vi "Constants.vi"   [LabVIEW 2017, in "DSF Core.lvlib"]
uses:
  DSF Core.lvlib
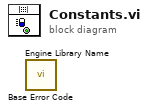
[diagram p0: block diagram]
diagram:
  n1 = call "Base Error Code.vi"() -> ()  [unwired: 11 in, 1 out]
  n2 = call "Engine Library Name.vi"() -> ()  [unwired: 11 in, 1 out]
